vi "PH_ImageCalibrator.Draw Image.vi"(0 "i ref in":refnum<vi>, 2 "Cam Image":T1, 5 "error in (no error)":errorcluster) -> (14 "i ref out":refnum<vi>, 19 "error out":errorcluster)   [LabVIEW 2014, in "PH_ImageCalibrator.lvlib"]
doc: "This VI draws the image to the GUI. Depending on the sequencer state, it writes the images also to the attributes or calculates the pixel sum."
uses:
  PH_ImageCalibrator.lvlib
  <vilib>/vision/Image Controls.llb/IMAQ Image.ctl
  CS_Core/BaseSM/BaseSM.lvlib
  CS_Core/BaseProcess/BaseProcess.lvlib
  PH_Basics/PH_Img_BaseClass/PH_Img_BaseClass.lvlib
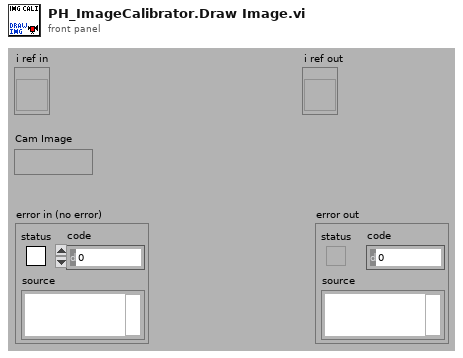
[diagram p1: front panel]
types:
  T1 = typedef "IMAQ Image.ctl" = refnum<image>
  T2 = typedef "PH_Img_BaseClass.lvlib/PH_Img_BaseClass.i attribute.ctl" = cluster{"GUI Refs":T3, "Timeout Image [ms]":i32, "Default Periodic Period [ms]":i32, "Camera":cluster{"Instancename":string, "Notifier":refnum<notifier>}, "Palette":T4, "Cam Settings":cluster{"Cam ID":string, "Gain":dbl, "Brightness":dbl, "Shutter":dbl, "Cam Info Failure":bool, "Mode":i32}}
  T3 = typedef "PH_Img_BaseClass.lvlib/PH_Img_BaseClass.GUI Refs.ctl" = cluster{"Timeout":refnum<vi>, "Image":refnum<vi>, "Palette":refnum<vi>, "Timeout Set":refnum<vi>}
  T4 = typedef "PH_Img_BaseClass.lvlib/PH_Img_BaseClass.Palette.ctl" = i32
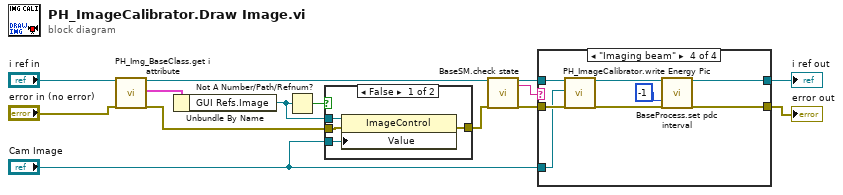
[diagram p0: block diagram]
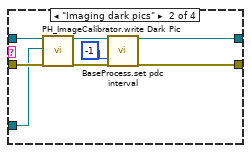
[diagram p4: hidden frame]
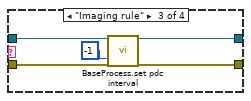
[diagram p5: hidden frame]
diagram:
  n1 = call "PH_Img_BaseClass.get i attribute.vi"("i ref in"="i ref in", "error in (no error)"="error in (no error)") -> ("i ref out"=w7:refnum<vi>, "i attribute"=w5:T2, "error out"=w2:errorcluster)  [unwired: 15 in]
  n2 = Unbundle By Name(w5) -> ("GUI Refs.Image"=w3:refnum<vi>)
  n3 = Not A Number/Path/Refnum?(number/path/refnum=w3) -> (NaN/Path/Refnum?=w4:bool)
  n4 = case shown="False" w4 {
    tunnel: w3 -> [w18 _]
    tunnel: [w17 w19] -> w8
    tunnel: w2 -> [w16 w19]
    tunnel: "Cam Image" -> [w15 _]
    frame False {
      n5 = property class="ImageControl"(reference=w18, error in=w16, "Value"=w15) -> (error out=w17:errorcluster)  [unwired: 1 out]
    }
    frame True {
    }
  }
  n6 = call "BaseSM.check state.vi"("i ref in"=w7, "error in (no error)"=w8) -> ("i ref out"=w10:refnum<vi>, "actualState"=w9:string, "error out"=w11:errorcluster)  [unwired: 12 in, 3 out]
  n7 = case shown="\"Imaging beam\"" w9 {
    tunnel: [w20 w23 w32 w40] -> w12
    tunnel: w11 -> [w20 w29 w30 w39]
    tunnel: w10 -> [w21 w28 w31 w38]
    tunnel: [w21 w25 w33 w41] -> w14
    tunnel: "Cam Image" -> [_ w22 _ w37]
    frame Default {
    }
    frame "Imaging dark pics" {
      n8 = call "PH_ImageCalibrator.write Dark Pic.vi"("i ref in"=w28, "Cam Image"=w22, "error in (no error)"=w29) -> ("i ref out"=w26:refnum<vi>, "error out"=w24:errorcluster)  [unwired: 15 in]
      n9 = call "BaseProcess.set pdc interval.vi"("i ref in"=w26, "PeriodicInterval [ms]"=-1 ("PeriodicInterval"), "error in (no error)"=w24) -> ("i ref out"=w25:refnum<vi>, "error out"=w23:errorcluster)  [unwired: 14 in, 1 out]
    }
    frame "Imaging rule" {
      n10 = call "BaseProcess.set pdc interval.vi"("i ref in"=w31, "PeriodicInterval [ms]"=-1 ("PeriodicInterval"), "error in (no error)"=w30) -> ("i ref out"=w33:refnum<vi>, "error out"=w32:errorcluster)  [unwired: 14 in, 1 out]
    }
    frame "Imaging beam" {
      n11 = call "PH_ImageCalibrator.write Energy Pic.vi"("i ref in"=w38, "Cam Image"=w37, "error in (no error)"=w39) -> ("i ref out"=w35:refnum<vi>, "error out"=w36:errorcluster)  [unwired: 15 in]
      n12 = call "BaseProcess.set pdc interval.vi"("i ref in"=w35, "PeriodicInterval [ms]"=-1 ("PeriodicInterval"), "error in (no error)"=w36) -> ("i ref out"=w41:refnum<vi>, "error out"=w40:errorcluster)  [unwired: 14 in, 1 out]
    }
  }
  "error out" <- w12
  "i ref out" <- w14
